vi "send_sms.vi"(6 "error in (no error)":errorcluster, 10 "message":string, 11 "mobile phone email":string) -> (0 "error out":errorcluster, 2 "standard output":string, 3 "standard error":string)   [LabVIEW 2012]
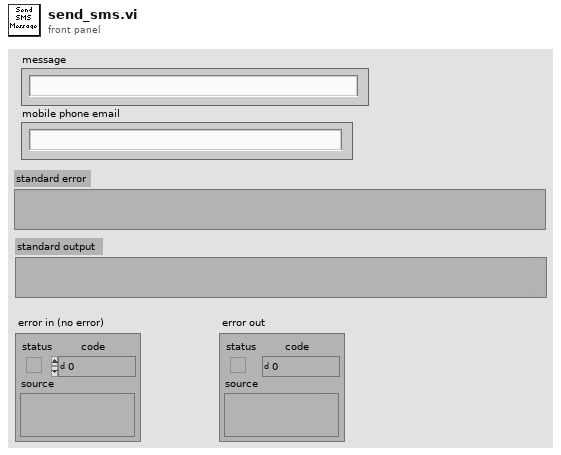
[diagram p1: front panel]
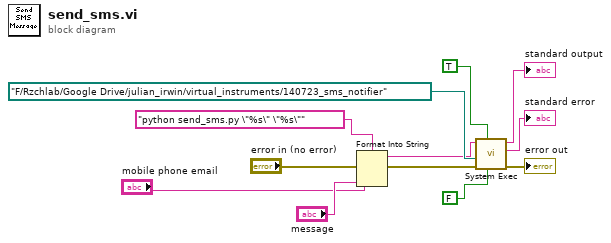
[diagram p0: block diagram]
diagram:
  n1 = Format Into String(format string="python send_sms.py \"%s\" \"%s\"" ("command line"), error in="error in (no error)", "mobile phone email", "message") -> (resulting string=w3:string, error out=w4:errorcluster)  [unwired: 1 in]
  n2 = call <vilib>:"System Exec.vi"("run minimized? (F)"=FALSE, "wait until completion? (T)"=TRUE, "error in (no error)"=w4, "working directory"=path "F:/Rzchlab/Google Drive/julian_irwin/virtual_instruments/140723_sms_notifier", "command line"=w3) -> ("error out"=→"error out":errorcluster, "standard error"=→"standard error":string, "standard output"=→"standard output":string)  [unwired: 3 in, 1 out]
